vi "Configure Gating Center Span.vi"(7 "Span Time (2E-9 s)":dbl=2e-09, 8 "error in (no error)":errorcluster, 9 "Center Time (0 s)":dbl, 10 "Channel (1)":i32=1, 11 "VISA resource name":refnum<visa-resource-name>) -> (0 "error out":errorcluster, 3 "VISA resource name out":refnum<visa-resource-name>)   [LabVIEW 2018, in "Keysight PNA Series.lvlib"]
doc: "Configures the gate filter span time and center time."
uses:
  Keysight PNA Series.lvlib
panel:
  # "TODO:\nSpan Time has problem."
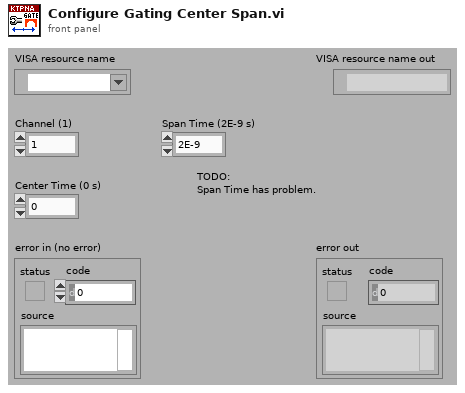
[diagram p1: front panel]
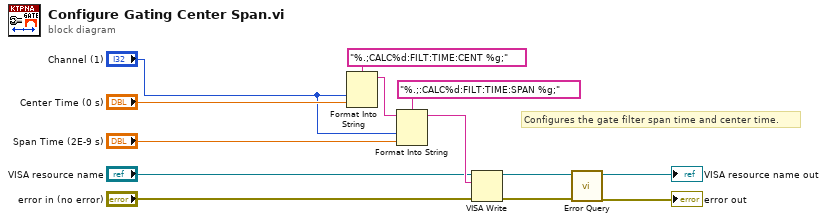
[diagram p0: block diagram]
diagram:
  # "Configures the gate filter span time and center time."
  n1 = Format Into String(format string="%.;CALC%d:FILT:TIME:CENT %g;", "Channel (1)", "Center Time (0 s)") -> (resulting string=w11:string)  [unwired: 2 in, 1 out]
  n2 = Format Into String(format string="%.;:CALC%d:FILT:TIME:SPAN %g;", initial string=w11, "Channel (1)", "Span Time (2E-9 s)") -> (resulting string=w9:string)  [unwired: 1 in, 1 out]
  n3 = VISA Write(VISA resource name="VISA resource name", write buffer=w9, error in (no error)="error in (no error)") -> (VISA resource name out=w6:refnum<visa-resource-name>, error out=w5:errorcluster)  [unwired: 1 out]
  n4 = call "Error Query.vi"("error in (no error)"=w5, "VISA resource name"=w6) -> ("error out"=→"error out":errorcluster, "VISA resource name out"=→"VISA resource name out":refnum<visa-resource-name>)  [unwired: 6 in, 2 out]
